vi "_FPGA_AmplitudeModulation.vi"(7 "Amplitude(0-16384)":u16 max=16384 step=1, 10 "Input":fxp<+,14,14>) -> (2 "Output":fxp<+,14,14>)   [LabVIEW 2018]
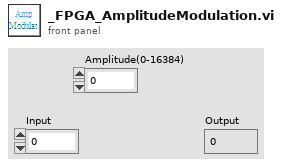
[diagram p1: front panel]
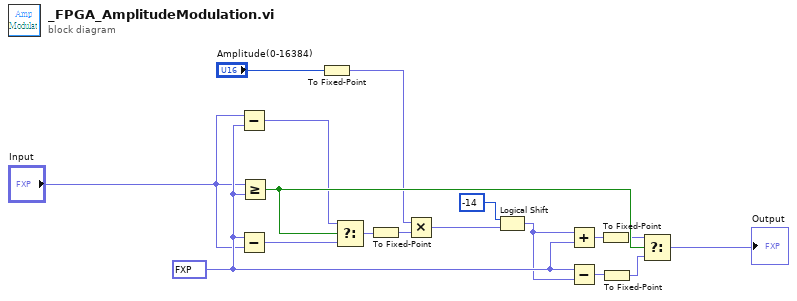
[diagram p0: block diagram]
diagram:
  w14 = fxp<+,15,15> 8192.0 ("y")
  n1 = Subtract(x="Input", y=w14) -> (x-y=w12:fxp<+/-,16,16>)
  n2 = Subtract(x=w14, y="Input") -> (x-y=w11:fxp<+/-,16,16>)
  n3 = Greater Or Equal?(x="Input", y=w14) -> (x >= y?=w13:bool)
  n4 = To Fixed-Point(number="Amplitude(0-16384)") -> (fixed-point=w2:fxp<+,16,16>)  [unwired: 1 in]
  n5 = Select(t=w12, s=w13, f=w11) -> (s? t:f=w9:fxp<+/-,16,16>)
  n6 = To Fixed-Point(number=w9) -> (fixed-point=w8:fxp<+,14,14>)  [unwired: 1 in]
  n7 = Multiply(x=w2, y=w8) -> (x*y=w15:fxp<+,30,30>)
  n8 = Logical Shift(y=-14 ("index"), x=w15) -> (x << y=w10:fxp<+,30,30>)
  n9 = Add(x=w10, y=w14) -> (x+y=w5:fxp<+,31,31>)
  n10 = Subtract(x=w14, y=w10) -> (x-y=w7:fxp<+/-,31,31>)
  n11 = To Fixed-Point(number=w5) -> (fixed-point=w4:fxp<+,14,14>)  [unwired: 1 in]
  n12 = To Fixed-Point(number=w7) -> (fixed-point=w6:fxp<+,14,14>)  [unwired: 1 in]
  n13 = Select(t=w4, s=w13, f=w6) -> (s? t:f=→"Output":fxp<+,14,14>)
